vi "Create IHandlePublished.vi"(8 "error in":errorcluster, 11 "IWampMessage":refnum<class "IWampMessage.lvclass">) -> (0 "error out":errorcluster, 3 "IHandlePublished":refnum<class "IHandlePublished.lvclass">)   [LabVIEW 2020, in "wamplv.lvlib"]
uses:
  wamplv.lvlib
  SerialisedMessages/JSONMessage/WampMessage JSON.lvclass
  SerialisedMessages/IWampMessage/IWampMessage.lvclass
  SerialisedMessages/MsgPackMessage/WampMessage MsgPack.lvclass
  HandlePublished JSON/HandlePublished JSON.lvclass
  HandlePublished MsgPack/HandlePublished MsgPack.lvclass
  C:/local/wamplv/Private/Requests/IGenericInternalMessage/IGenericInternalMessage.lvclass
  C:/local/wamplv/Private/Requests/IInternalMessage/IInternalMessage.lvclass
  C:/local/wamplv/Private/Requests/MessageReceivedHandlers/HandlePublished/IHandlePublished/IHandlePublished.lvclass
  C:/local/wamplv/Private/Requests/MessageReceivedHandlers/HandlePublished/HandlePublished JSON/HandlePublished JSON.lvclass
  C:/local/wamplv/Private/Requests/MessageReceivedHandlers/IJsonMessageHandler/IJsonMessageHandler.lvclass
  C:/local/wamplv/Private/Requests/MessageReceivedHandlers/HandlePublished/HandlePublished MsgPack/HandlePublished MsgPack.lvclass
  C:/local/wamplv/Private/Requests/MessageReceivedHandlers/IMsgPackMessageHandler/IMsgPackMessageHandler.lvclass
  IHandlePublished/IHandlePublished.lvclass
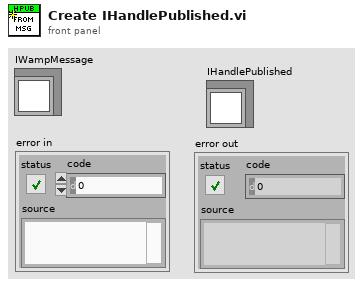
[diagram p1: front panel]
types:
  T1 = typedef "wamplv.lvlib/WAMP Client.lvclass/Serialisation.ctl" = enum16{"JSON", "MessagePack"}
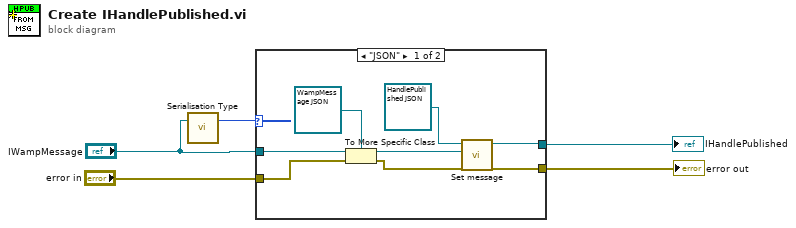
[diagram p0: block diagram]
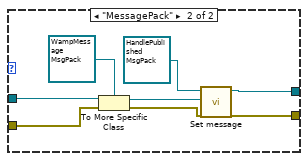
[diagram p2: hidden frame]
diagram:
  n1 = call-dynamic "Serialisation Type.vi"("IWampMessage in"="IWampMessage") -> ("Serialisation Type"=w5:T1)  [unwired: 2 in]
  n2 = case shown="\"JSON\"" w5 {
    tunnel: "IWampMessage" -> [w12 w19]
    tunnel: "error in" -> [w10 w18]
    tunnel: [w8 w16] -> w2
    tunnel: [w6 w13] -> w1
    frame "JSON" {
      n3 = To More Specific Class(target class=refnum<class "WampMessage JSON.lvclass"> refnum ("wamplv.lvlib:JSONMessage.lvclass"), reference=w12, error in=w10) -> (specific class reference=w7:refnum<class "WampMessage JSON.lvclass">, error out=w6:errorcluster)
      n4 = call-dynamic "Set message.vi"("WampMessage JSON"=w7, "IMsgPackMessageHandler in"=refnum<class "HandlePublished JSON.lvclass"> refnum ("wamplv.lvlib:HandlePublished JSON.lvclass")) -> ("IMsgPackMessageHandler out"=w8:refnum<class "HandlePublished JSON.lvclass">)  [unwired: 9 in]
    }
    frame "MessagePack" {
      n5 = To More Specific Class(target class=refnum<class "WampMessage MsgPack.lvclass"> refnum ("wamplv.lvlib:MsgPackMessage.lvclass"), reference=w19, error in=w18) -> (specific class reference=w15:refnum<class "WampMessage MsgPack.lvclass">, error out=w13:errorcluster)
      n6 = call-dynamic "Set message.vi"("WampMessage MsgPack"=w15, "HandlePublished MsgPack in"=refnum<class "HandlePublished MsgPack.lvclass"> refnum ("wamplv.lvlib:HandlePublished MsgPack.lvclass")) -> ("HandlePublished MsgPack out"=w16:refnum<class "HandlePublished MsgPack.lvclass">)  [unwired: 9 in]
    }
  }
  "IHandlePublished" <- w2
  "error out" <- w1
